vi "2.2.vi"() -> ()   [LabVIEW 2017]
uses:
  sin.vi
panel:
  in  "停止":bool
  out "波形图表 共享":dbl(graph)
  out "波形图表 全局":dbl(graph)
  # "任务二"
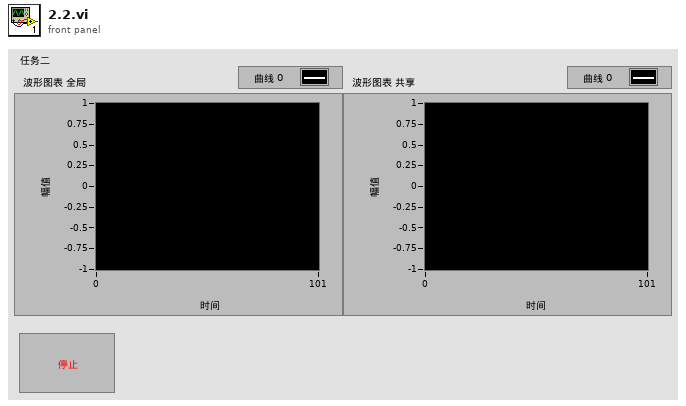
[diagram p1: front panel]
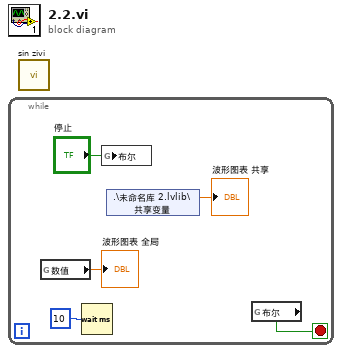
[diagram p0: block diagram]
diagram:
  n1 = while {
    stop <- w3 stop-if-true
    n2 = global read "sin.vi" "数值"() -> (→"波形图表 全局":dbl)
    n3 = Wait (ms)(milliseconds to wait=10) -> ()  [unwired: 1 out]
    n4 = global write "sin.vi" "布尔"("停止") -> ()
    n5 = shared-variable ".\\未命名库 2.lvlib\\共享变量"() -> (→"波形图表 共享":dbl)  [unwired: 1 in, 1 out]
    n6 = global read "sin.vi" "布尔"() -> (w3:bool)
  }
  n7 = call "sin zivi.vi"() -> ()  [unwired: 12 in]
